vi "Parse_control_array.vi"(1 "Messreihe":i32) -> ()   [LabVIEW 2019]
uses:
  Global Variables/global.vi
  Global Variables/Data_Display_global.vi
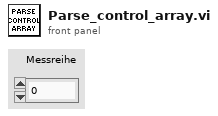
[diagram p1: front panel]
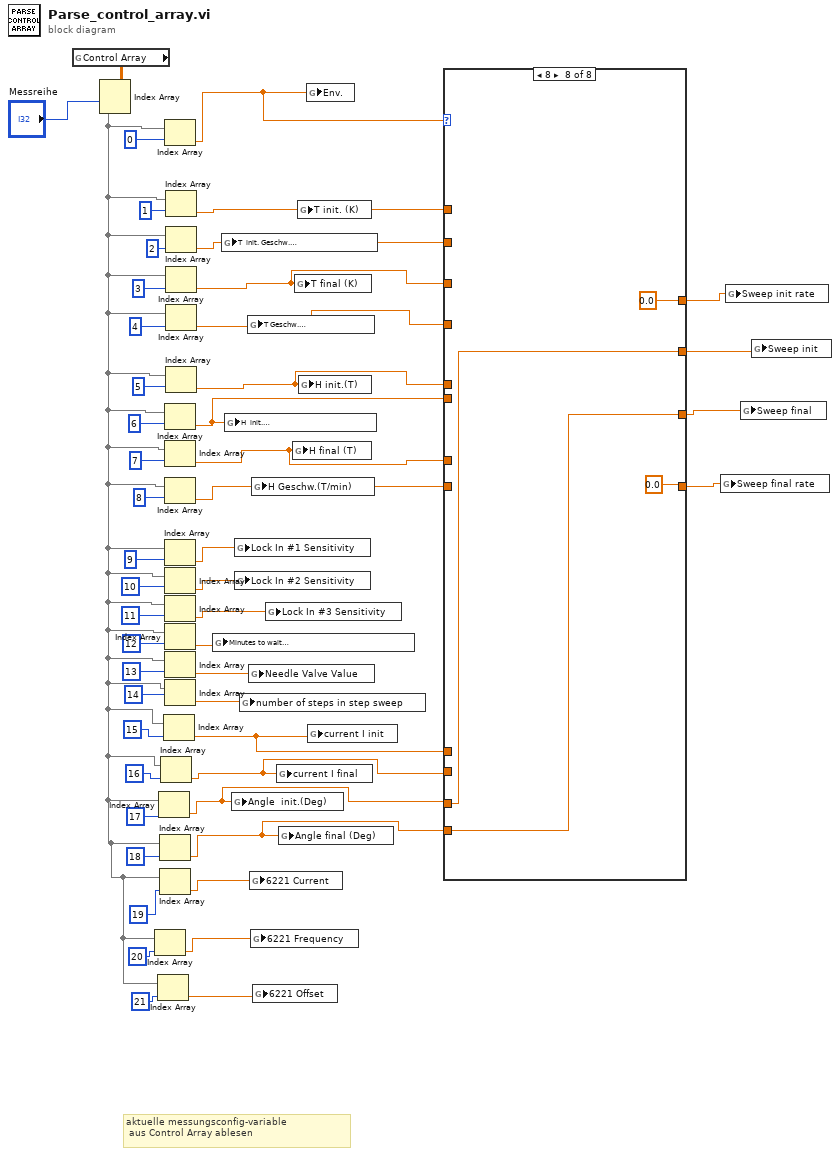
[diagram p0: block diagram]
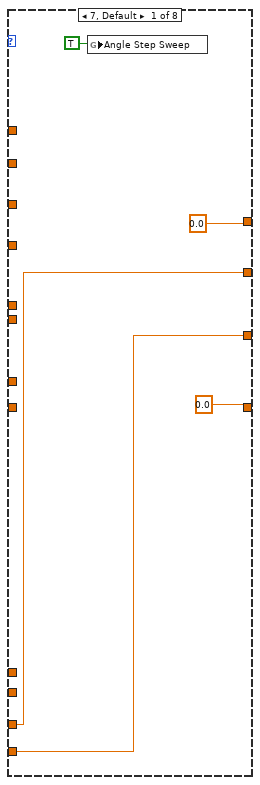
[diagram p2: hidden frame]
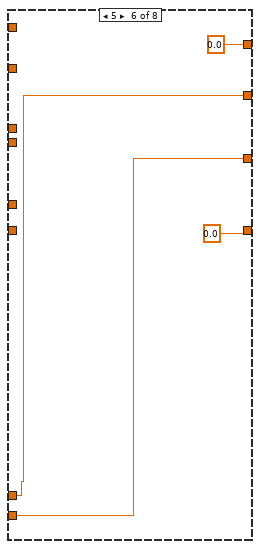
[diagram p7: hidden frame]
diagram:
  # "aktuelle messungsconfig-variable\n aus Control Array ablesen"
  n1 = global read "global.vi" "Control Array"() -> (w51:dbl[][])
  n2 = Index Array(array=w51, index (row)="Messreihe") -> (element=w10:dbl[])  [unwired: 1 in]
  n3 = Index Array(array=w10, index=20) -> (element=w2:dbl)
  n4 = Index Array(array=w10, index=21) -> (element=w1:dbl)
  n5 = Index Array(array=w10, index=17) -> (element=w5:dbl)
  n6 = Index Array(array=w10, index=18) -> (element=w4:dbl)
  n7 = Index Array(array=w10, index=19) -> (element=w3:dbl)
  n8 = Index Array(array=w10, index=16) -> (element=w6:dbl)
  n9 = Index Array(array=w10, index=15) -> (element=w7:dbl)
  n10 = Index Array(array=w10, index=0) -> (element=w26:dbl)
  n11 = Index Array(array=w10, index=6) -> (element=w15:dbl)
  n12 = Index Array(array=w10, index=7) -> (element=w22:dbl)
  n13 = Index Array(array=w10, index=8) -> (element=w14:dbl)
  n14 = Index Array(array=w10, index=9) -> (element=w34:dbl)
  n15 = Index Array(array=w10, index=10) -> (element=w33:dbl)
  n16 = Index Array(array=w10, index=11) -> (element=w32:dbl)
  n17 = Index Array(array=w10, index=12) -> (element=w31:dbl)
  n18 = Index Array(array=w10, index=13) -> (element=w9:dbl)
  n19 = Index Array(array=w10, index=14) -> (element=w8:dbl)
  n20 = Index Array(array=w10, index=1) -> (element=w25:dbl)
  n21 = Index Array(array=w10, index=2) -> (element=w12:dbl)
  n22 = Index Array(array=w10, index=3) -> (element=w24:dbl)
  n23 = Index Array(array=w10, index=4) -> (element=w11:dbl)
  n24 = Index Array(array=w10, index=5) -> (element=w23:dbl)
  n25 = global write "global.vi" "Minutes to wait\nafter initialization"(w31) -> ()
  n26 = global write "global.vi" "T  init. Geschw. \n(K/min)"(w12) -> ()
  n27 = global write "global.vi" "H  init. \nGeschw.(T/min)"(w15) -> ()
  n28 = global write "global.vi" "Angle  init.(Deg)"(w5) -> ()
  n29 = global write "global.vi" "Lock In #1 Sensitivity"(w34) -> ()
  n30 = global write "global.vi" "Lock In #2 Sensitivity"(w33) -> ()
  n31 = global write "global.vi" "number of steps in step sweep"(w8) -> ()
  n32 = global write "global.vi" "T Geschw. \n(K/min)"(w11) -> ()
  n33 = global write "global.vi" "Needle Valve Value"(w9) -> ()
  n34 = global write "global.vi" "6221 Current"(w3) -> ()
  n35 = global write "global.vi" "6221 Frequency"(w2) -> ()
  n36 = global write "global.vi" "H Geschw.(T/min)"(w14) -> ()
  n37 = global write "global.vi" "6221 Offset"(w1) -> ()
  n38 = global write "global.vi" "Lock In #3 Sensitivity"(w32) -> ()
  n39 = global write "global.vi" "current I final"(w6) -> ()
  n40 = global write "global.vi" "Angle final (Deg)"(w4) -> ()
  n41 = global write "global.vi" "H final (T)"(w22) -> ()
  n42 = global write "global.vi" "T final (K)"(w24) -> ()
  n43 = global write "global.vi" "T init. (K)"(w25) -> ()
  n44 = global write "global.vi" "H init.(T)"(w23) -> ()
  n45 = global write "global.vi" "Env."(w26) -> ()
  n46 = global write "global.vi" "current I init"(w7) -> ()
  n47 = case shown="8" w26 {
    tunnel: w25 -> [_ _ w64 w68 _ _ w80 _]
    tunnel: w24 -> [_ _ w63 _ _ _ _ _]
    tunnel: w23 -> [_ w60 _ _ w72 _ w79 _]
    tunnel: w22 -> [_ w59 _ w67 w71 _ _ _]
    tunnel: w6 -> [_ _ _ _ _ w76 _ _]
    tunnel: w5 -> [w55 _ _ _ _ _ _ w84]
    tunnel: w4 -> [w54 _ _ _ _ _ _ w83]
    tunnel: [w55 w60 w64 w68 w72 w73 w80 w84] -> w21
    tunnel: [w54 w59 w63 w67 w71 w76 w79 w83] -> w20
    tunnel: [0.0 w58 w62 w66 w70 0.0 w78 0.0] -> w16
    tunnel: w15 -> [_ w58 _ _ w70 _ _ _]
    tunnel: w14 -> [_ w57 _ _ w69 _ _ _]
    tunnel: [0.0 w57 w61 w65 w69 0.0 w77 0.0] -> w13
    tunnel: w12 -> [_ _ w62 w66 _ _ w78 _]
    tunnel: w11 -> [_ _ w61 w65 _ _ w77 _]
    tunnel: w7 -> [_ _ _ _ _ w73 _ _]
    frame 7, Default {
      n48 = global write "Data_Display_global.vi" "Angle Step Sweep"(TRUE) -> ()
    }
    frame 1 {
    }
    frame 2 {
    }
    frame 3 {
    }
    frame 4 {
    }
    frame 5 {
    }
    frame 6 {
    }
    frame 8 {
    }
  }
  n49 = global write "global.vi" "Sweep final rate"(w13) -> ()
  n50 = global write "global.vi" "Sweep init rate"(w16) -> ()
  n51 = global write "global.vi" "Sweep final"(w20) -> ()
  n52 = global write "global.vi" "Sweep init"(w21) -> ()
